vi "MoveStone.vi"(0 "Chessboard":T1, 5 "ItemIndex":T2, 7 "StoneColor":u16, 11 "error in (no error)":errorcluster) -> (4 "output array":T1, 8 "StoneColor out":u16, 15 "error out":errorcluster)   [LabVIEW 2009]
doc: "Move stone on the certain index position."
uses:
  Controls/Chess.ctl
  Controls/ItemIndex.ctl
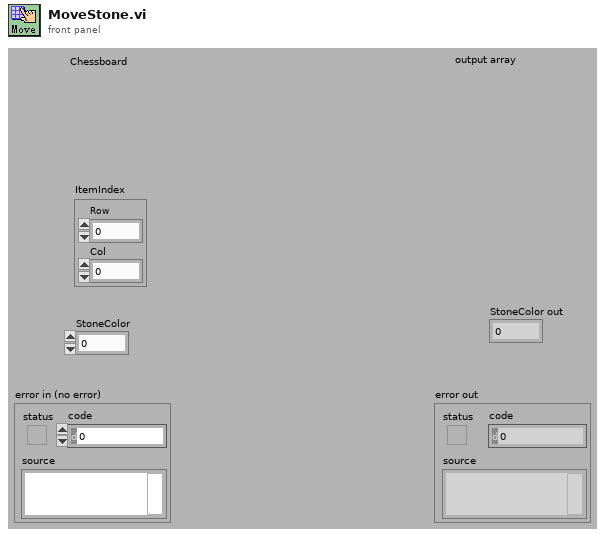
[diagram p1: front panel]
types:
  T1 = typedef "Chess.ctl" = u16[][]
  T2 = typedef "ItemIndex.ctl" = cluster{"Row":i32, "Col":i32}
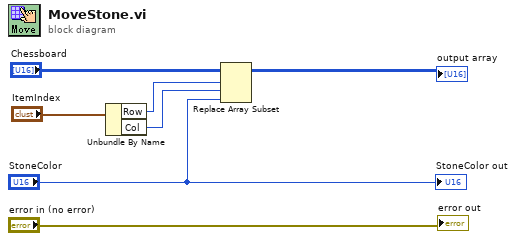
[diagram p0: block diagram]
diagram:
  n1 = Unbundle By Name("ItemIndex") -> ("Row"=w5:i32, "Col"=w4:i32)
  n2 = Replace Array Subset(array="Chessboard", new element="StoneColor", index (row)=w5, index (col)=w4) -> (→"output array":T1)
  "error out" <- "error in (no error)"
  "StoneColor out" <- "StoneColor"
